vi "editActuator.vi"(10 "Actuator":T1={"Serial Configurations for Sensors"={"Motor Temperature Sensor"={"VISA resource name"="", "Baud Rate"=9600, "Data Bits"=8, "Parity"=enum."None", "Stop Bits"=10, "Flow Control"=0, "Timeout (ms)"=10000, "Serial Protocol"=enum."RS485"}, "Ambient Temperature Sensor"={"VISA resource name"="", "Baud Rate"=9600, "Data Bits"=8, "Parity"=enum."None", "Stop Bits"=10, "Flow Control"=0, "Timeout (ms)"=10000, "Serial Protocol"=enum."RS485"}, "Distance Gauge"={"VISA resource name"="", "Baud Rate"=9600, "Data Bits"=8, "Parity"=enum."None", "Stop Bits"=10, "Flow Control"=0, "Timeout (ms)"=10000, "Serial Protocol"=enum."RS485"}}, "Stepper Motor"={"Maximum Step Rate"=5000000.0}, "Sensor Data"={"Force Sensor Conversion"=100.0}, "Controller"={"Per Step Delta Force"=5000.0}, "Exception Stop Conditions"={"Motor Overheat Temperature"=274.15}} {"Exception Stop Conditions"."Motor Overheat Temperature" min=274.15 max=573.15 format="%.1f"; "Controller"."Per Step Delta Force" min=10.0 max=5000.0; "Sensor Data"."Force Sensor Conversion" min=0.01 max=5000.0 format="%.2f"; "Stepper Motor"."Maximum Step Rate" min=10000.0 max=5000000.0; "Serial Configurations for Sensors"."Distance Gauge"."Stop Bits" items=["1.0"=10, "1.5"=15, "2.0"=20]; "Serial Configurations for Sensors"."Distance Gauge"."Flow Control" items=["None", "XON/XOFF", "RTS/CTS", "XON/XOFF & RTS/CTS", "DTR/DSR", "XON/XOFF & DTR/DSR"]; "Serial Configurations for Sensors"."Distance Gauge"."Data Bits" min=5 max=8 step=1; "Serial Configurations for Sensors"."Ambient Temperature Sensor"."Stop Bits" items=["1.0"=10, "1.5"=15, "2.0"=20]; "Serial Configurations for Sensors"."Ambient Temperature Sensor"."Flow Control" items=["None", "XON/XOFF", "RTS/CTS", "XON/XOFF & RTS/CTS", "DTR/DSR", "XON/XOFF & DTR/DSR"]; "Serial Configurations for Sensors"."Ambient Temperature Sensor"."Data Bits" min=5 max=8 step=1; "Serial Configurations for Sensors"."Motor Temperature Sensor"."Stop Bits" items=["1.0"=10, "1.5"=15, "2.0"=20]; "Serial Configurations for Sensors"."Motor Temperature Sensor"."Flow Control" items=["None", "XON/XOFF", "RTS/CTS", "XON/XOFF & RTS/CTS", "DTR/DSR", "XON/XOFF & DTR/DSR"]; "Serial Configurations for Sensors"."Motor Temperature Sensor"."Data Bits" min=5 max=8 step=1}) -> (1 "canceledIsTrue":bool=TRUE, 2 "Actuator 2":T1={"Serial Configurations for Sensors"={"Motor Temperature Sensor"={"VISA resource name"="", "Baud Rate"=9600, "Data Bits"=8, "Parity"=enum."None", "Stop Bits"=10, "Flow Control"=0, "Timeout (ms)"=10000, "Serial Protocol"=enum."RS485"}, "Ambient Temperature Sensor"={"VISA resource name"="", "Baud Rate"=9600, "Data Bits"=8, "Parity"=enum."None", "Stop Bits"=10, "Flow Control"=0, "Timeout (ms)"=10000, "Serial Protocol"=enum."RS485"}, "Distance Gauge"={"VISA resource name"="", "Baud Rate"=9600, "Data Bits"=8, "Parity"=enum."None", "Stop Bits"=10, "Flow Control"=0, "Timeout (ms)"=10000, "Serial Protocol"=enum."RS485"}}, "Stepper Motor"={"Maximum Step Rate"=5000000.0}, "Sensor Data"={"Force Sensor Conversion"=100.0}, "Controller"={"Per Step Delta Force"=5000.0}, "Exception Stop Conditions"={"Motor Overheat Temperature"=274.15}} {"Exception Stop Conditions"."Motor Overheat Temperature" min=274.15 max=573.15 format="%.1f"; "Controller"."Per Step Delta Force" min=10.0 max=5000.0; "Sensor Data"."Force Sensor Conversion" min=0.01 max=5000.0 format="%.2f"; "Stepper Motor"."Maximum Step Rate" min=10000.0 max=5000000.0; "Serial Configurations for Sensors"."Distance Gauge"."Stop Bits" items=["1.0"=10, "1.5"=15, "2.0"=20]; "Serial Configurations for Sensors"."Distance Gauge"."Flow Control" items=["None", "XON/XOFF", "RTS/CTS", "XON/XOFF & RTS/CTS", "DTR/DSR", "XON/XOFF & DTR/DSR"]; "Serial Configurations for Sensors"."Distance Gauge"."Data Bits" min=5 max=8 step=1; "Serial Configurations for Sensors"."Ambient Temperature Sensor"."Stop Bits" items=["1.0"=10, "1.5"=15, "2.0"=20]; "Serial Configurations for Sensors"."Ambient Temperature Sensor"."Flow Control" items=["None", "XON/XOFF", "RTS/CTS", "XON/XOFF & RTS/CTS", "DTR/DSR", "XON/XOFF & DTR/DSR"]; "Serial Configurations for Sensors"."Ambient Temperature Sensor"."Data Bits" min=5 max=8 step=1; "Serial Configurations for Sensors"."Motor Temperature Sensor"."Stop Bits" items=["1.0"=10, "1.5"=15, "2.0"=20]; "Serial Configurations for Sensors"."Motor Temperature Sensor"."Flow Control" items=["None", "XON/XOFF", "RTS/CTS", "XON/XOFF & RTS/CTS", "DTR/DSR", "XON/XOFF & DTR/DSR"]; "Serial Configurations for Sensors"."Motor Temperature Sensor"."Data Bits" min=5 max=8 step=1})   [LabVIEW 2013]
uses:
  Configuration/Actuator.ctl
  Configuration/Serial Configuration For Sensors.ctl
  <userlib>/Common/SerialProtocols/Configuration/SerialConfig.ctl
  <userlib>/Common/SerialProtocols/Configuration/SerialProtocol.ctl
  Configuration/Stepper Motor.ctl
  Configuration/SensorData.ctl
  Configuration/Compensator.ctl
  Configuration/Exception Stop Conditions.ctl
  <userlib>/Common/SerialProtocols/SerialProtocols.lvlib
panel:
  in  "CancelIsTrue":bool
  in  "OKIsTrue":bool
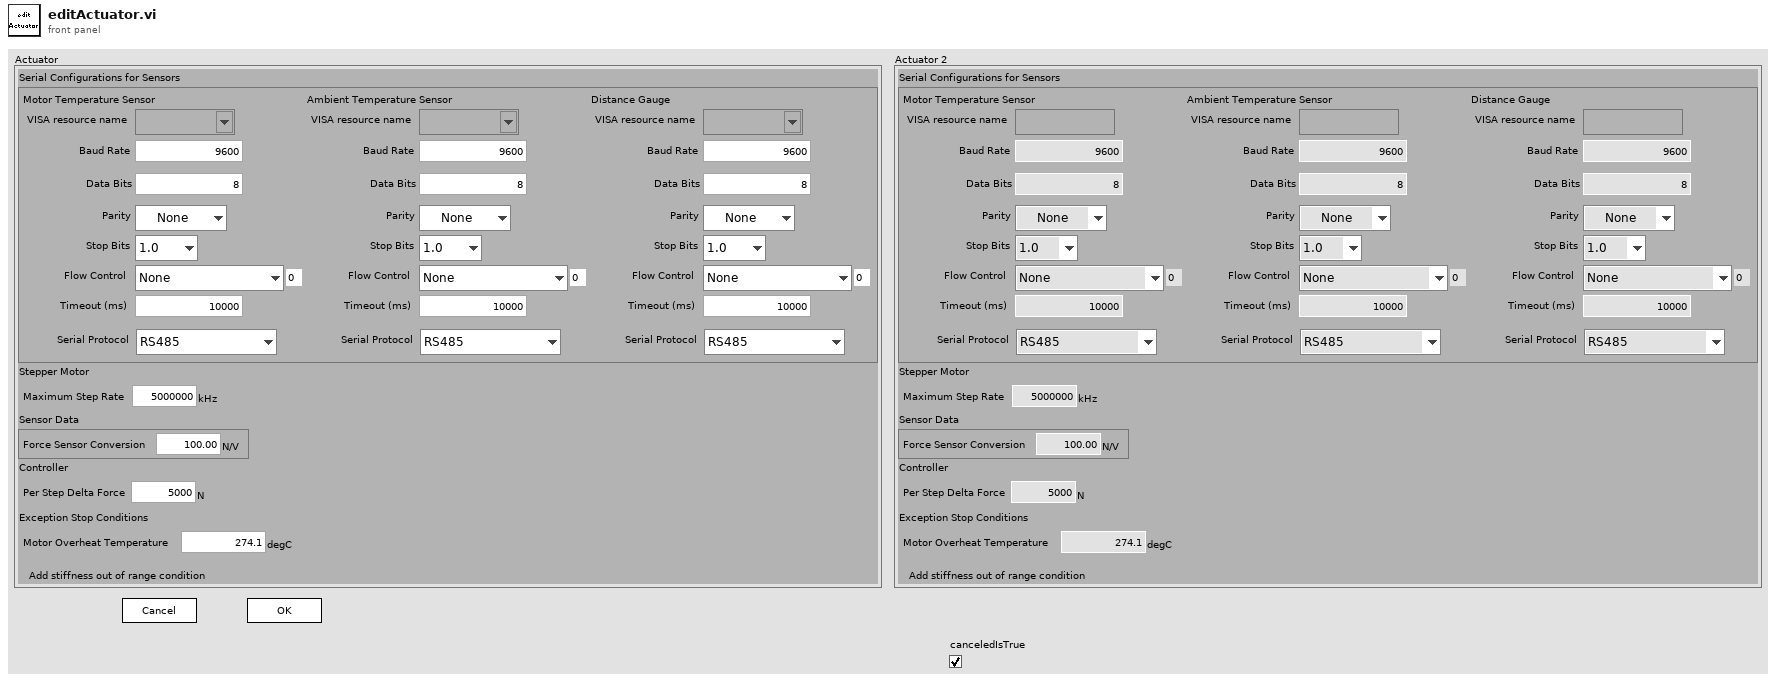
[diagram p1: front panel]
types:
  T1 = typedef "Actuator.ctl" = cluster{"Serial Configurations for Sensors":T2, "Stepper Motor":T5, "Sensor Data":T6, "Controller":T7, "Exception Stop Conditions":T8}
  T2 = typedef "Serial Configuration For Sensors.ctl" = cluster{"Motor Temperature Sensor":T3, "Ambient Temperature Sensor":T3, "Distance Gauge":T3}
  T3 = typedef "SerialProtocols.lvlib/SerialConfig.ctl" = cluster{"VISA resource name":refnum<visa-resource-name>, "Baud Rate":u32, "Data Bits":u16, "Parity":enum16{"None", "Odd", "Even", "Mark", "Space"}, "Stop Bits":u16, "Flow Control":u16, "Timeout (ms)":u32, "Serial Protocol":T4}
  T4 = typedef "SerialProtocols.lvlib/SerialProtocol.ctl" = enum16{"RS232", "RS485", "SerialSimulator"}
  T5 = typedef "Stepper Motor.ctl" = cluster{"Maximum Step Rate":dbl[unit]}
  T6 = typedef "SensorData.ctl" = cluster{"Force Sensor Conversion":dbl[unit]}
  T7 = typedef "Compensator.ctl" = cluster{"Per Step Delta Force":dbl[unit]}
  T8 = typedef "Exception Stop Conditions.ctl" = cluster{"Motor Overheat Temperature":dbl[unit]}
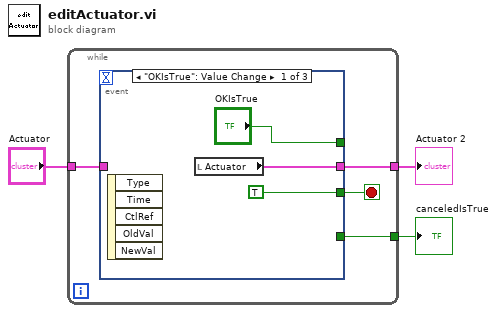
[diagram p0: block diagram]
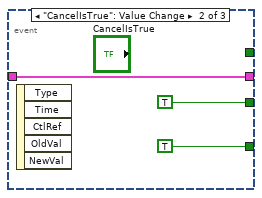
[diagram p2: hidden frame]
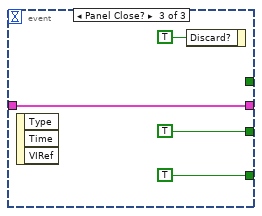
[diagram p3: hidden frame]
diagram:
  n1 = while {
    tunnel: [w7] -> w3
    tunnel: [w6] -> w2
    tunnel: "Actuator" -> [w5]
    stop <- w4 stop-if-true
    n2 = event shown="[0] \"OKIsTrue\": Value Change" {
      selector: _ -> [_ _ _]
      dyn-events: _ -> [_ _ _]
      timeout: _ -> [_ _ _]
      tunnel: ["OKIsTrue" _ _] -> _
      tunnel: [_ TRUE ("Discard?") TRUE ("Discard?")] -> w7
      tunnel: [w9 w12 w15] -> w6
      tunnel: w5 -> [_ w12 w15]
      tunnel: [TRUE TRUE TRUE] -> w4
      event "OKIsTrue": Value Change {
        n3 = event-data() -> ()  [unwired: 1 in, 5 out]
        n4 = local read "Actuator"() -> (w9:T1)
      }
      event "CancelIsTrue": Value Change {
        n5 = event-data() -> ()  [unwired: 1 in, 5 out]
      }
      event Panel Close? {
        n6 = event-data() -> ()  [unwired: 1 in, 3 out]
        n7 = event-data("Discard?"=TRUE) -> ()  [unwired: 1 in, 1 out]
      }
    }
  }
  "canceledIsTrue" <- w3
  "Actuator 2" <- w2
